vi "ReadyState.vi"(8 "error in (no error)":errorcluster, 10 "Player":refnum<class "Player.lvclass">, 11 "ReadyState in":refnum<class "ReadyState.lvclass">) -> (0 "error out":errorcluster, 3 "ReadyState out":refnum<class "ReadyState.lvclass">)   [LabVIEW 2017, in "ReadyState.lvclass"]
uses:
  ReadyState.lvclass
  Player Class/Player.lvclass
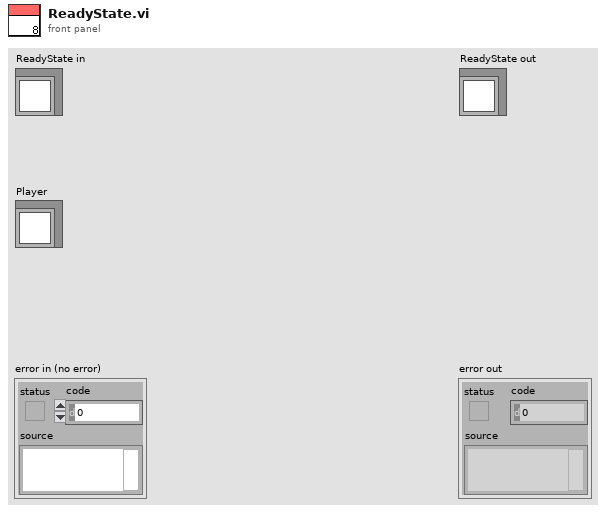
[diagram p1: front panel]
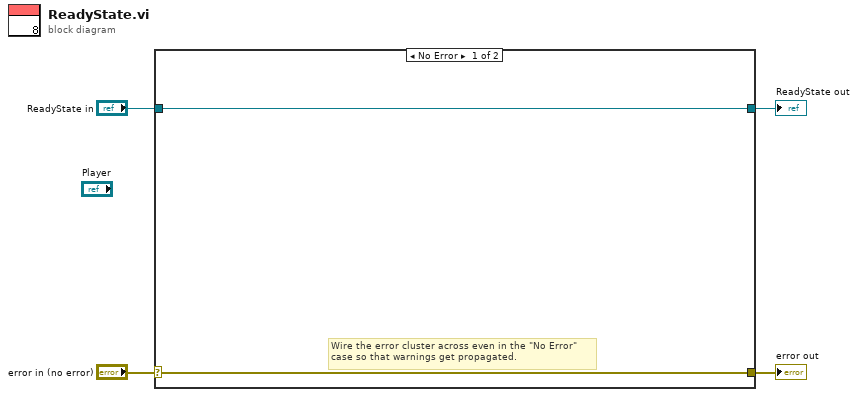
[diagram p0: block diagram]
diagram:
  n1 = case shown="No Error" "error in (no error)" {
    selector: "error in (no error)" -> [w6 w8]
    tunnel: [w6 w8] -> w3
    tunnel: [w5 w7] -> w1
    tunnel: "ReadyState in" -> [w5 w7]
    frame No Error {
      # "Wire the error cluster across even in the \"No Error\"\ncase so that warnings get propagated."
    }
    frame Error {
    }
  }
  "error out" <- w3
  "ReadyState out" <- w1
